vi "Set Gas.vi"(8 "error in":errorcluster, 10 "Gas":T1, 11 "Alicat Device in":refnum<class "Alicat Device.lvclass">) -> (0 "error out":errorcluster, 2 "DataOut":string, 3 "Alicat Device out":refnum<class "Alicat Device.lvclass">)   [LabVIEW 2014, in "Alicat Lib.lvlib" / "Alicat Device.lvclass"]
doc: "Set the gas that the device uses to run it's calculations."
uses:
  Alicat Device.lvclass
  Controls/Gas.ctl
  Alicat Device.lvclass/Alicat Device.ctl
  reusable/Session APIs/Serial/Public/Get Data/Get String.vi
  reusable/Session APIs/Serial/Serial Session.lvclass
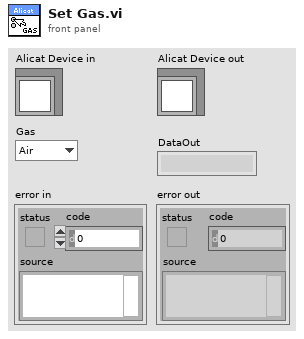
[diagram p1: front panel]
types:
  T1 = typedef "Alicat Lib.lvlib/Alicat Device.lvclass/Gas.ctl" = enum16{"Air", "Ar", "CH4", "CO", "CO2", "C2H6", "H2", "He", "N2", "NO", "Ne", "O2", "C3H8", "n-C4H10", "C2H2", "C2H4", "i-C2H10", "Kr", "Xe"}
  T2 = typedef "Serial Session.lvclass/Session Handle.ctl" = refnum<data-value>
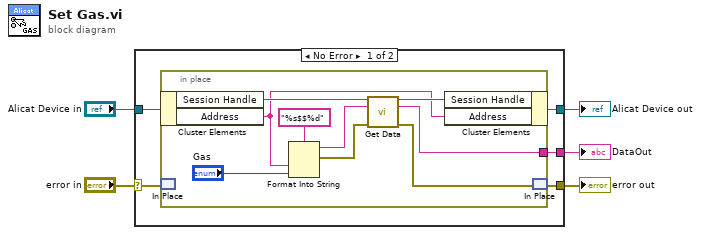
[diagram p0: block diagram]
diagram:
  n1 = case shown="No Error" "error in" {
    selector: "error in" -> [w10 w21]
    tunnel: [w8 w21] -> w4
    tunnel: [w6 w20] -> w2
    tunnel: "Alicat Device in" -> [w7 w20]
    tunnel: [w9 _] -> w1
    frame No Error {
      n2 = in-place {
        in-place-border: [w17] -> w9
        n3 = in-place-cluster #1(w7) -> ("Session Handle"=w19:T2, "Address"=w14:string)
        n4 = in-place-match #2(w10) -> ()  [unwired: 1 out]
        n5 = Format Into String(format string="%s$$%d", w14, "Gas") -> (resulting string=w13:string, error out=w12:errorcluster)  [unwired: 2 in]
        n6 = call-poly "Get Data.vi"("Session Handle in"=w19, "CMD"=w13, "error in"=w12) -> ("Session Handle out"=w18:T2, "DataOut"=w17:string, "error out"=w16:errorcluster)  [unwired: 10 in]
        n7 = in-place-cluster #1("Session Handle"=w18, "Address"=w14) -> (w6:refnum<class "Alicat Device.lvclass">)
        n8 = in-place-match #2(w16) -> (w8:errorcluster)
      }
    }
    frame Error {
    }
  }
  "error out" <- w4
  "Alicat Device out" <- w2
  "DataOut" <- w1
